vi "Load Bitfile.vi"() -> ()   [LabVIEW 2011]
uses:
  vi.lib/LabVIEW Hacker/Adept/Private/Type Defs/Adept Device Ctl.xctl
  vi.lib/LabVIEW Hacker/Adept/LVH-Adept.lvlib
  <vilib>/LabVIEW Hacker/LVH-Toolbox/Common/LVH-Common.lvlib
panel:
  out "Status":string
  out "Error Out":errorcluster
  in  "Stop Button":bool
  in  "Program Button":bool
  in  "Bit File Path":path
  in  "Adept Device":u16(xcontrol)
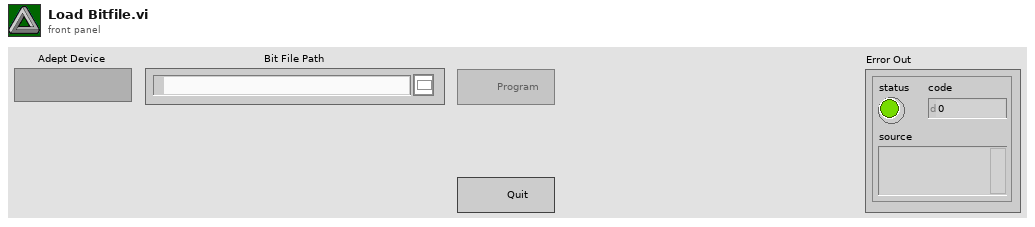
[diagram p1: front panel]
types:
  T1 = enum8{"Enabled", "Disabled", "Disabled and Grayed Out"}
  T2 = typedef "LVH-Adept.lvlib/Device Config.ctl" = cluster{"Num Devices":i32, "Device Names":string[], "Device Index":u16, "Device Handle":u32, "Status":T3}
  T3 = typedef "LVH-Adept.lvlib/Status.ctl" = cluster{"DEPP":bool, "DSTM":bool, "DJTG":bool}
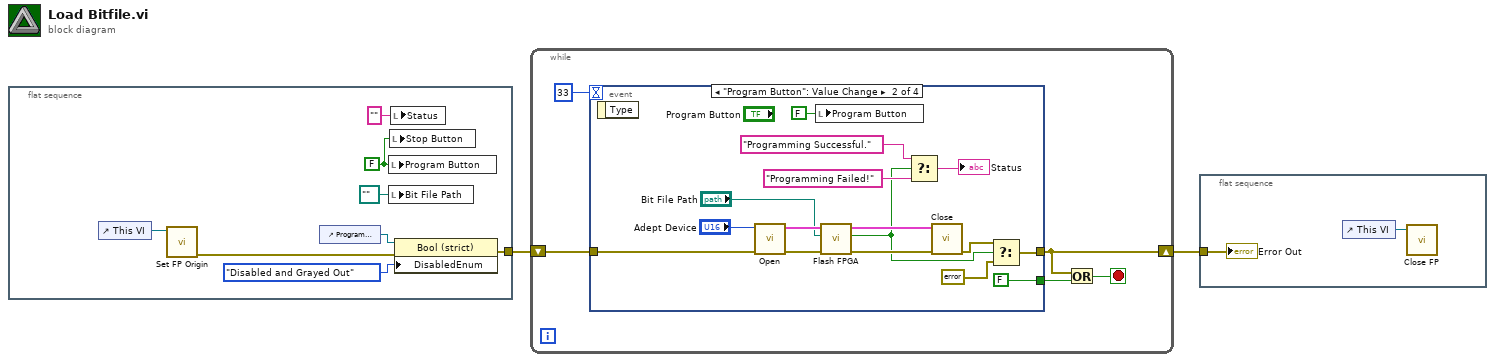
[diagram p0: block diagram]
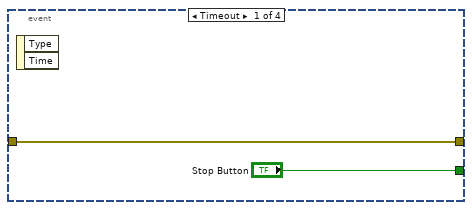
[diagram p2: hidden frame]
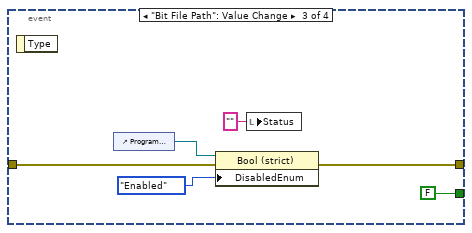
[diagram p3: hidden frame]
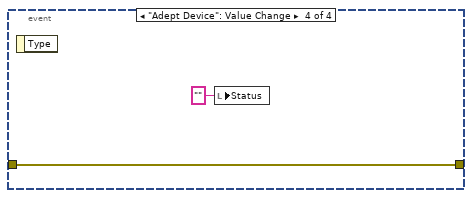
[diagram p4: hidden frame]
diagram:
  n1 = flat-sequence {
    tunnel: [w9] -> w2
    frame #0 {
      w6 = FALSE ("Program Button")
      n2 = control-ref of="This VI"() -> (w3:refnum<vi>)
      n3 = call <vilib>:"Set FP Origin.vi"("VI Ref"=w3) -> ("Error Out"=w4:errorcluster)  [unwired: 10 in]
      n4 = control-ref of="Program Button"() -> (w7:refnum<vi>)
      n5 = local write "Program Button"(w6) -> ()
      n6 = local write "Bit File Path"(path "" ("Bit File Path")) -> ()
      n7 = local write "Stop Button"(w6) -> ()
      n8 = local write "Status"("" ("Status")) -> ()
      n9 = property class="Bool (strict)"(reference=w7, error in=w4, "DisabledEnum"=T1."Disabled and Grayed Out" ("Disabled")) -> (error out=w9:errorcluster)  [unwired: 1 out]
    }
  }
  n10 = while {
    shift-right: [w13] -> w1
    shift-left: w2 -> [w14]
    stop <- w12 stop-if-true
    n11 = event shown="[1] \"Program Button\": Value Change" {
      selector: _ -> [_ _ _ _]
      dyn-events: _ -> [_ _ _ _]
      timeout: 33 -> [_ _ _ _]
      tunnel: w14 -> [w16 w26 w37 w40]
      tunnel: [w16 w20 w38 w40] -> w13
      tunnel: ["Stop Button" FALSE ("Stop Button") FALSE ("Stop Button") _] -> w11
      event Timeout {
        n12 = event-data() -> ()  [unwired: 1 in, 2 out]
      }
      event "Program Button": Value Change {
        n13 = event-data() -> ()  [unwired: 1 in, 1 out]
        n14 = call "Open.vi"("Error In"=w26, "Adept Device"="Adept Device") -> ("Error Out"=w31:errorcluster, "Adept Config"=w32:T2)  [unwired: 8 in]
        n15 = local write "Program Button"(FALSE ("Program Button")) -> ()
        n16 = call "Flash FPGA.vi"("Error In"=w31, "Bit File Path"="Bit File Path", "Adept Config"=w32) -> ("Error Out"=w30:errorcluster, "Success?"=w21:bool, "Adept Config"=w29:T2)  [unwired: 6 in]
        n17 = Select(t="Programming Successful.", s=w21, f="Programming Failed!") -> (s? t:f=→"Status":string)
        n18 = call "Close.vi"("Error In"=w30, "Adept Config"=w29) -> ("Error Out"=w19:errorcluster)  [unwired: 9 in]
        n19 = Select(t=w19, s=w21, f=errorcluster {"status"=FALSE, "code"=0, "source"=""}) -> (s? t:f=w20:errorcluster)
      }
      event "Bit File Path": Value Change {
        n20 = event-data() -> ()  [unwired: 1 in, 1 out]
        n21 = control-ref of="Program Button"() -> (w35:refnum<vi>)
        n22 = property class="Bool (strict)"(reference=w35, error in=w37, "DisabledEnum"=T1."Enabled" ("Disabled")) -> (error out=w38:errorcluster)  [unwired: 1 out]
        n23 = local write "Status"("" ("Status")) -> ()
      }
      event "Adept Device": Value Change {
        n24 = event-data() -> ()  [unwired: 1 in, 1 out]
        n25 = local write "Status"("" ("Status")) -> ()
      }
    }
    n26 = Or(x=w13, y=w11) -> (x .or. y?=w12:bool)
  }
  n27 = flat-sequence {
    tunnel: w1 -> [w42]
    frame #0 {
      n28 = control-ref of="This VI"() -> (w43:refnum<vi>)
      n29 = call <vilib>:"Close FP.vi"("VI Ref"=w43) -> ()  [unwired: 10 in, 1 out]
      "Error Out" <- w42
    }
  }
